vi "Exit.vi"(8 "error in (no error)":errorcluster, 11 "Old State":refnum<class "Manual.lvclass">) -> (0 "error out":errorcluster, 3 "New State":refnum<class "Manual.lvclass">)   [LabVIEW 2014, in "States.lvlib" / "Manual.lvclass"]
doc: "This is an abstract method. Override this method to define the behavior when you leave the state."
uses:
  Manual.lvclass
  <vilib>/ActorFramework/Message Enqueuer/Message Enqueuer.lvclass/Message Enqueuer.ctl
  <vilib>/ActorFramework/Message Enqueuer/Enqueue.vi
  <vilib>/ActorFramework/Message Priority Queue/Priority Enqueue.vi
  Process State/CoordinatorState.lvclass
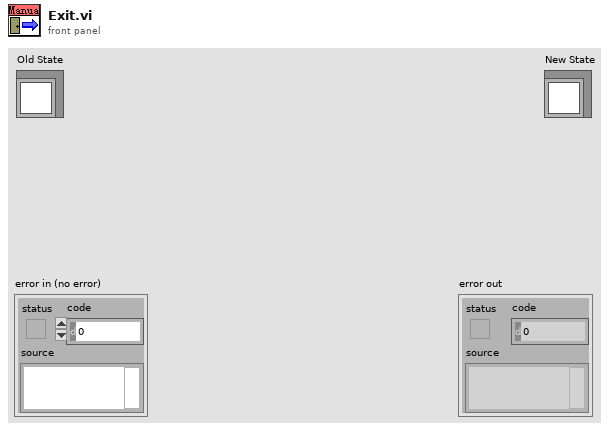
[diagram p1: front panel]
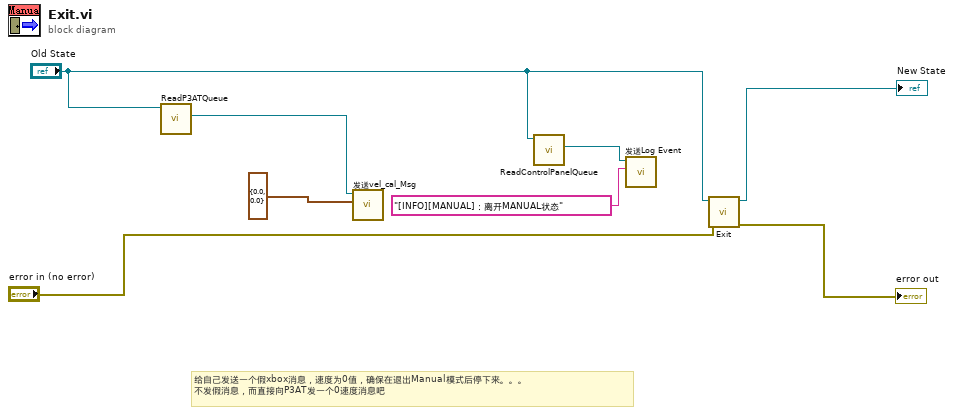
[diagram p0: block diagram]
diagram:
  # "给自己发送一个假xbox消息，速度为0值，确保在退出Manual模式后停下来。。。\n不发假消息，而直接向P3AT发一个0速度消息吧"
  n1 = call-dynamic "ReadP3ATQueue.vi"("CoordinatorState输入"="Old State") -> ("操作者框架:消息待入队列"=w5:refnum<class "Message Enqueuer.lvclass">)  [unwired: 8 in, 2 out]
  n2 = call "发送vel_cal_Msg.vi"("值(信号)"=cluster{"rot_z":dbl, "lin_x":dbl} {"rot_z"=0.0, "lin_x"=0.0}, "消息待入队列"=w5) -> ()  [unwired: 8 in, 2 out]
  n3 = call-dynamic "ReadControlPanelQueue.vi"("CoordinatorState输入"="Old State") -> ("操作者框架:消息待入队列"=w3:refnum<class "Message Enqueuer.lvclass">)  [unwired: 8 in, 2 out]
  n4 = call "发送Log Event.vi"("Event Text"="[INFO][MANUAL]：离开MANUAL状态", "消息待入队列"=w3) -> ()  [unwired: 8 in, 2 out]
  n5 = call-parent "Exit.vi"("error in (no error)"="error in (no error)", "Old State"="Old State") -> ("error out"=→"error out":errorcluster, "New State"=→"New State":refnum<class "Manual.lvclass">)  [unwired: 8 in]
